vi "SW_Save_parameter_group_2.vi"(7 "Researcher name":string="Researcher", 8 "error in":errorcluster, 9 "Settings cluster in":T1={"Defaults"={"Default User"=0.0, "VISA Resource Name "="Tracker"}, "Recording and saving"={"Researcher name"="Researcher", "Name prefix"="Track", "Data post-processing"={"Filter type"=enum."Savitzky-Golay", "Length"=31, "Order"=3}, "Stop at"=0.0, "\"Stop at\" enabled"=FALSE, "Default save folder path"=path "", "Acquisition FPS"=enum."Max"}, "Geometry"={"Cage diameter, mm"=180, "Starting angle MIDFIELD"=0, "Starting angle BORDER"=0, "Radius, mm CENTER"=30, "Radius, mm MIDFIELD"=75, "N segments MIDFIELD"=2, "N segments BORDER"=4, "R-gap, mm"=0.0, "Bridge swap"=FALSE, "Bridge H. offset"=0.0, "Bridge V. offset"=0.0, "Twisted neck"=FALSE, "Alt. magn. orientation"=FALSE}, "IO parameters"={"IO general config."=12, "IO 1 configuration"=1, "IO 2 configuration"=1, "IO 3 configuration"=0, "IO 4 configuration"=0, "Activate ext. RS-232"=0, "IO inversion config."=0, "Sync capability"=1}, "Stimulus presets array"=[{"Event type"=0, "Dur., s"=0.0, "Stim., s"=0.0, "TTL out N"=1, "Set/Clear"=FALSE, "Stim. has been set"=FALSE}, {"Event type"=0, "Dur., s"=0.0, "Stim., s"=0.0, "TTL out N"=1, "Set/Clear"=FALSE, "Stim. has been set"=FALSE}, {"Event type"=0, "Dur., s"=0.0, "Stim., s"=0.0, "TTL out N"=1, "Set/Clear"=FALSE, "Stim. has been set"=FALSE}, {"Event type"=0, "Dur., s"=0.0, "Stim., s"=0.0, "TTL out N"=1, "Set/Clear"=FALSE, "Stim. has been set"=FALSE}, {"Event type"=0, "Dur., s"=0.0, "Stim., s"=0.0, "TTL out N"=1, "Set/Clear"=FALSE, "Stim. has been set"=FALSE}, {"Event type"=0, "Dur., s"=0.0, "Stim., s"=0.0, "TTL out N"=1, "Set/Clear"=FALSE, "Stim. has been set"=FALSE}, {"Event type"=0, "Dur., s"=0.0, "Stim., s"=0.0, "TTL out N"=1, "Set/Clear"=FALSE, "Stim. has been set"=FALSE}, {"Event type"=0, "Dur., s"=0.0, "Stim., s"=0.0, "TTL out N"=1, "Set/Clear"=FALSE, "Stim. has been set"=FALSE}, {"Event type"=0, "Dur., s"=0.0, "Stim., s"=0.0, "TTL out N"=1, "Set/Clear"=FALSE, "Stim. has been set"=FALSE}, {"Event type"=0, "Dur., s"=0.0, "Stim., s"=0.0, "TTL out N"=1, "Set/Clear"=FALSE, "Stim. has been set"=FALSE}, {"Event type"=0, "Dur., s"=0.0, "Stim., s"=0.0, "TTL out N"=1, "Set/Clear"=FALSE, "Stim. has been set"=FALSE}, {"Event type"=0, "Dur., s"=0.0, "Stim., s"=0.0, "TTL out N"=1, "Set/Clear"=FALSE, "Stim. has been set"=FALSE}, {"Event type"=0, "Dur., s"=0.0, "Stim., s"=0.0, "TTL out N"=1, "Set/Clear"=FALSE, "Stim. has been set"=FALSE}, {"Event type"=0, "Dur., s"=0.0, "Stim., s"=0.0, "TTL out N"=1, "Set/Clear"=FALSE, "Stim. has been set"=FALSE}], "Calibration parameters"={"Timing calibration sw/hw"=1.0, "True FPS"=80.0, "True frame time, s"=0.0125, "Disp. calibration info"=[]}, "Settings loaded OK"=FALSE} {"Calibration parameters"."True frame time, s" format="%.10g"; "Calibration parameters"."Disp. calibration info"."Speed, µl per ms" format="%.3g"; "Calibration parameters"."True FPS" format="%.10g"; "Calibration parameters"."Timing calibration sw/hw" format="%.10g"; "Stimulus presets array"."Event type" items=["Stay for N seconds"]; "Stimulus presets array"."TTL out N" items=["1"=1, "2"=2, "1+2"=3]; "Recording and saving"."Data post-processing"."Order" min=3 max=11 step=2; "Recording and saving"."Data post-processing"."Length" min=5 max=301 step=2; "Geometry"."Cage diameter, mm" scale=0.0..340.0}, 10 "Parameter group":T9="Defaults", 11 "Settings file refnum in":T10) -> (0 "error out":errorcluster, 2 "Saved OK?":bool, 3 "Settings file refnum out":T10)   [LabVIEW 2018, in "Tracker.lvlib"]
uses:
  Tracker.lvlib
  <vilib>/Utility/config.llb/Config Data RefNum.ctl
  Controls/CTL_Settings_parameters_groups.ctl
  Controls/CTL_Settings_cluster.ctl
  Controls/CTL_Filter_selector.ctl
  Controls/CTL_Acquisition_speed_selector.ctl
  Controls/CTL_Segmented_plot_parameters.ctl
  Controls/CTL_IO_params_cluster.ctl
  Controls/CTL_Single_stimulus_setting.ctl
  Controls/CTL_Calibration_parameters.ctl
  Controls/CTL_Dispenser_calibration_info.ctl
  <vilib>/Utility/config.llb/NI_LVConfig.lvlib
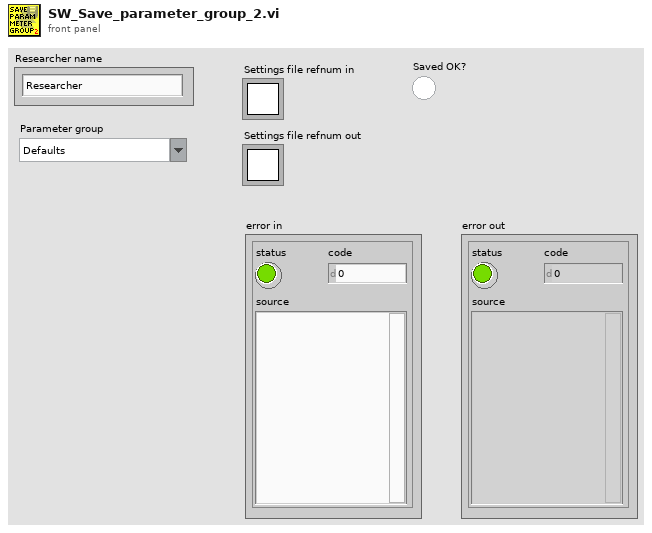
[diagram p1: front panel]
types:
  T1 = typedef "Tracker.lvlib/CTL_Settings_cluster.ctl" = cluster{"Defaults":cluster{"Default User":dbl, "VISA Resource Name ":string}, "Recording and saving":cluster{"Researcher name":string, "Name prefix":string, "Data post-processing":T2, "Stop at":dbl, "\"Stop at\" enabled":bool, "Default save folder path":path, "Acquisition FPS":T3}, "Geometry":T4, "IO parameters":T5, "Stimulus presets array":T6[], "Calibration parameters":T7, "Settings loaded OK":bool}
  T2 = typedef "Tracker.lvlib/CTL_Filter_selector.ctl" = cluster{"Filter type":enum16{"None", "Savitzky-Golay"}, "Length":i32, "Order":i32}
  T3 = typedef "Tracker.lvlib/CTL_Acquisition_speed_selector.ctl" = enum16{"Max", "Optimal", "Eco"}
  T4 = typedef "Tracker.lvlib/CTL_Segmented_plot_parameters.ctl" = cluster{"Cage diameter, mm":u16, "Starting angle MIDFIELD":i16, "Starting angle BORDER":i16, "Radius, mm CENTER":u16, "Radius, mm MIDFIELD":u16, "N segments MIDFIELD":u8, "N segments BORDER":u8, "R-gap, mm":sgl, "Bridge swap":bool, "Bridge H. offset":sgl, "Bridge V. offset":sgl, "Twisted neck":bool, "Alt. magn. orientation":bool}
  T5 = typedef "Tracker.lvlib/CTL_IO_params_cluster.ctl" = cluster{"IO general config.":u16, "IO 1 configuration":u16, "IO 2 configuration":u16, "IO 3 configuration":u16, "IO 4 configuration":u16, "Activate ext. RS-232":u16, "IO inversion config.":u16, "Sync capability":u8}
  T6 = typedef "Tracker.lvlib/CTL_Single_stimulus_setting.ctl" = cluster{"Event type":u16, "Dur., s":sgl, "Stim., s":sgl, "TTL out N":u16, "Set/Clear":bool, "Stim. has been set":bool}
  T7 = typedef "Tracker.lvlib/CTL_Calibration_parameters.ctl" = cluster{"Timing calibration sw/hw":dbl, "True FPS":dbl, "True frame time, s":dbl, "Disp. calibration info":T8}
  T8 = typedef "Tracker.lvlib/CTL_Dispenser_calibration_info.ctl" = cluster{"Channel":u8, "Speed, µl per ms":dbl}[]
  T9 = typedef "Tracker.lvlib/CTL_Settings_parameters_groups.ctl" = string
  T10 = typedef "NI_LVConfig.lvlib/Config Data RefNum.ctl" = refnum<k1>
  T11 = cluster{"Default User":dbl, "VISA Resource Name ":string}
  T12 = cluster{"Researcher name":string, "Name prefix":string, "Data post-processing":T2, "Stop at":dbl, "\"Stop at\" enabled":bool, "Default save folder path":path, "Acquisition FPS":T3}
  T13 = cluster{"Stimulus presets array[0]":T6, "Stimulus presets array[1]":T6, "Stimulus presets array[2]":T6, "Stimulus presets array[3]":T6, "Stimulus presets array[4]":T6, "Stimulus presets array[5]":T6, "Stimulus presets array[6]":T6, "Stimulus presets array[7]":T6, "Stimulus presets array[8]":T6, "Stimulus presets array[9]":T6, "Stimulus presets array[10]":T6, "Stimulus presets array[11]":T6, "Stimulus presets array[12]":T6, "Stimulus presets array[13]":T6}
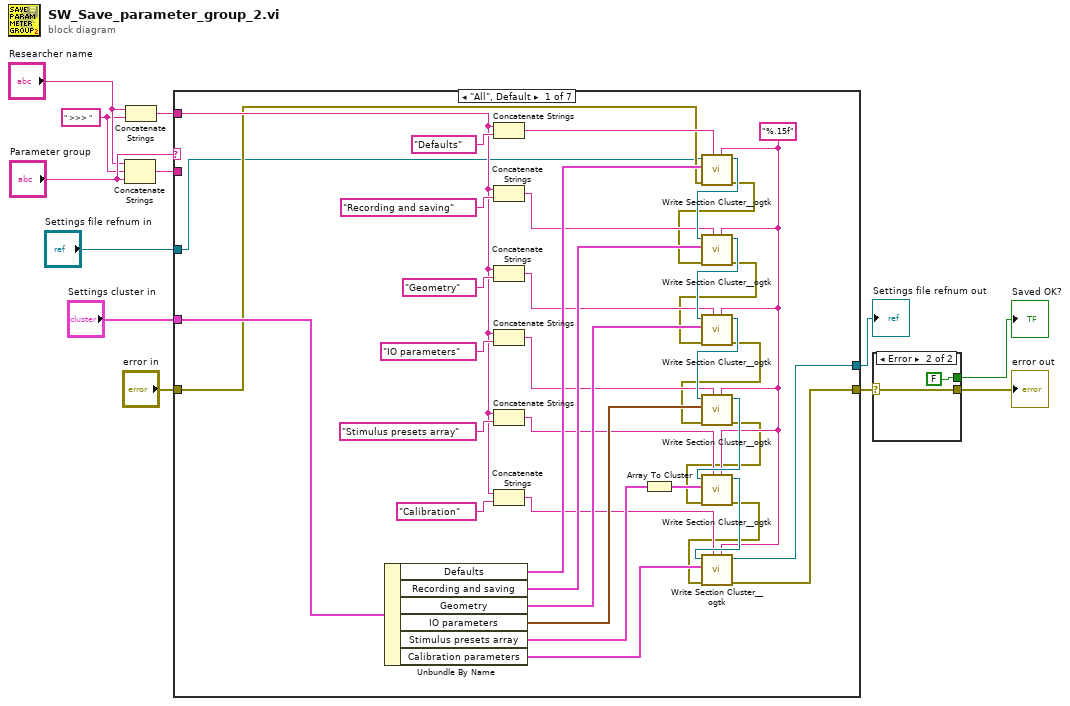
[diagram p0: block diagram]
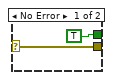
[diagram p2: hidden frame]
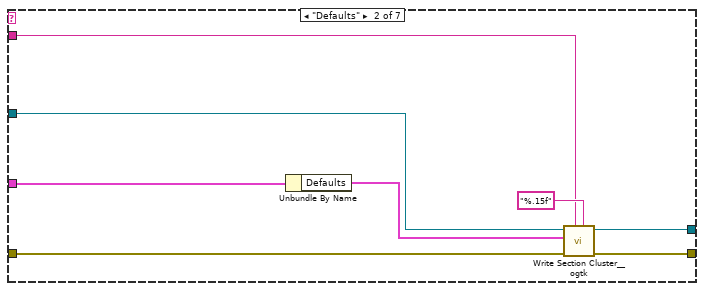
[diagram p3: hidden frame]
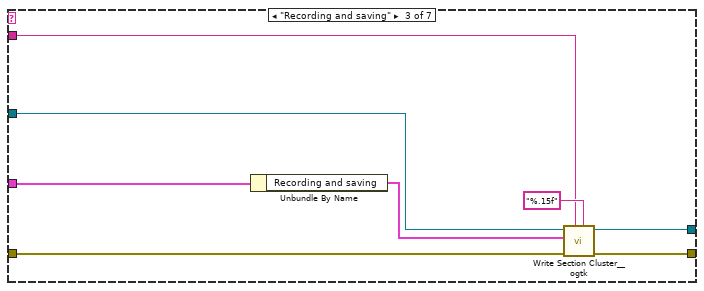
[diagram p4: hidden frame]
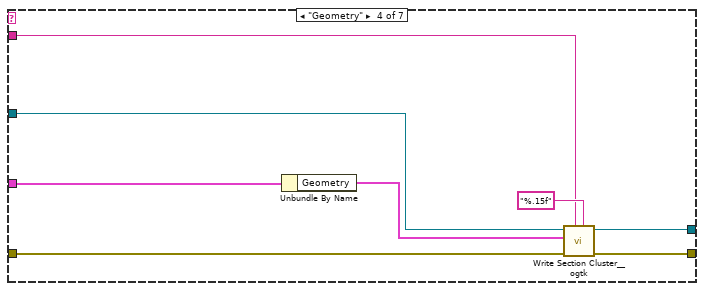
[diagram p5: hidden frame]
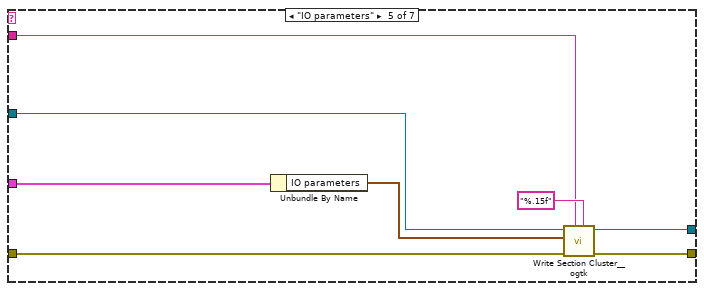
[diagram p6: hidden frame]
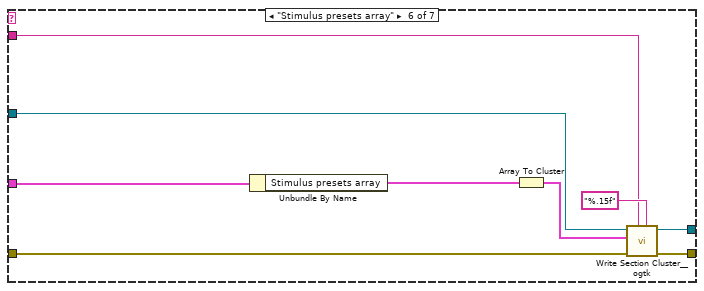
[diagram p7: hidden frame]
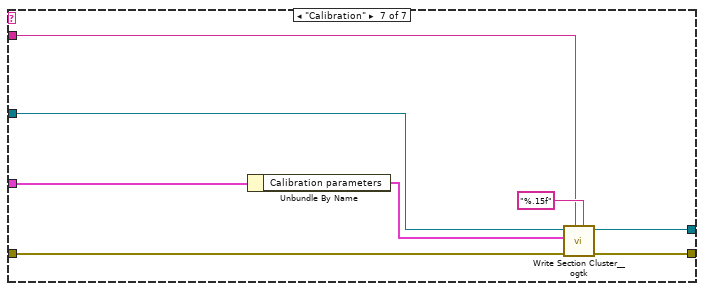
[diagram p8: hidden frame]
diagram:
  w2 = " >>> " ("string")
  n1 = Concatenate Strings("Researcher name", w2, "Parameter group") -> (w10:string)
  n2 = Concatenate Strings("Researcher name", w2) -> (w1:string)
  n3 = case shown="\"All\", Default" "Parameter group" {
    tunnel: "Settings cluster in" -> [w48 w54 w62 w70 w78 w87 w95]
    tunnel: w10 -> [_ w55 w63 w71 w79 w88 w96]
    tunnel: "error in" -> [w20 w53 w61 w69 w77 w86 w94]
    tunnel: "Settings file refnum in" -> [w19 w52 w60 w68 w76 w85 w93]
    tunnel: [w21 w51 w59 w67 w75 w84 w92] -> w8
    tunnel: [w13 w50 w58 w66 w74 w83 w91] -> w7
    tunnel: w1 -> [w24 _ _ _ _ _ _]
    frame "All", Default {
      w22 = "%.15f" ("float number format (optional)")
      n4 = Unbundle By Name(w48) -> ("Defaults"=w45:T11, "Recording and saving"=w41:T12, "Geometry"=w38:T4, "IO parameters"=w33:T5, "Stimulus presets array"=w28:T6[], "Calibration parameters"=w26:T7)
      n5 = Concatenate Strings(w24, T9 "Defaults" ("Parameter group")) -> (w47:string)
      n6 = Concatenate Strings(w24, T9 "Recording and saving" ("Parameter group")) -> (w42:string)
      n7 = Concatenate Strings(w24, T9 "Geometry" ("Parameter group")) -> (w37:string)
      n8 = Concatenate Strings(w24, T9 "IO parameters" ("Parameter group")) -> (w34:string)
      n9 = Concatenate Strings(w24, T9 "Stimulus presets array" ("Parameter group")) -> (w29:string)
      n10 = Concatenate Strings(w24, T9 "Calibration" ("Parameter group")) -> (w23:string)
      n11 = Array To Cluster(array=w28) -> (cluster=w27:T13)
      n12 = call <userlib>:"Write Section Cluster__ogtk.vi"("float number format (optional)"=w22, "section (optional)"=w47, "error in (no error)"=w20, "Section Formatted Cluster"=w45, "refnum"=w19) -> ("error out"=w18:errorcluster, "dup refnum"=w44:T10)  [unwired: 5 in]
      n13 = call <userlib>:"Write Section Cluster__ogtk.vi"("float number format (optional)"=w22, "section (optional)"=w42, "error in (no error)"=w18, "Section Formatted Cluster"=w41, "refnum"=w44) -> ("error out"=w17:errorcluster, "dup refnum"=w40:T10)  [unwired: 5 in]
      n14 = call <userlib>:"Write Section Cluster__ogtk.vi"("float number format (optional)"=w22, "section (optional)"=w37, "error in (no error)"=w17, "Section Formatted Cluster"=w38, "refnum"=w40) -> ("error out"=w16:errorcluster, "dup refnum"=w36:T10)  [unwired: 5 in]
      n15 = call <userlib>:"Write Section Cluster__ogtk.vi"("float number format (optional)"=w22, "section (optional)"=w34, "error in (no error)"=w16, "Section Formatted Cluster"=w33, "refnum"=w36) -> ("error out"=w15:errorcluster, "dup refnum"=w32:T10)  [unwired: 5 in]
      n16 = call <userlib>:"Write Section Cluster__ogtk.vi"("float number format (optional)"=w22, "section (optional)"=w29, "error in (no error)"=w15, "Section Formatted Cluster"=w27, "refnum"=w32) -> ("error out"=w14:errorcluster, "dup refnum"=w31:T10)  [unwired: 5 in]
      n17 = call <userlib>:"Write Section Cluster__ogtk.vi"("float number format (optional)"=w22, "section (optional)"=w23, "error in (no error)"=w14, "Section Formatted Cluster"=w26, "refnum"=w31) -> ("error out"=w13:errorcluster, "dup refnum"=w21:T10)  [unwired: 5 in]
    }
    frame "Defaults" {
      n18 = Unbundle By Name(w54) -> ("Defaults"=w49:T11)
      n19 = call <userlib>:"Write Section Cluster__ogtk.vi"("float number format (optional)"="%.15f", "section (optional)"=w55, "error in (no error)"=w53, "Section Formatted Cluster"=w49, "refnum"=w52) -> ("error out"=w50:errorcluster, "dup refnum"=w51:T10)  [unwired: 5 in]
    }
    frame "Recording and saving" {
      n20 = Unbundle By Name(w62) -> ("Recording and saving"=w57:T12)
      n21 = call <userlib>:"Write Section Cluster__ogtk.vi"("float number format (optional)"="%.15f", "section (optional)"=w63, "error in (no error)"=w61, "Section Formatted Cluster"=w57, "refnum"=w60) -> ("error out"=w58:errorcluster, "dup refnum"=w59:T10)  [unwired: 5 in]
    }
    frame "Geometry" {
      n22 = Unbundle By Name(w70) -> ("Geometry"=w65:T4)
      n23 = call <userlib>:"Write Section Cluster__ogtk.vi"("float number format (optional)"="%.15f", "section (optional)"=w71, "error in (no error)"=w69, "Section Formatted Cluster"=w65, "refnum"=w68) -> ("error out"=w66:errorcluster, "dup refnum"=w67:T10)  [unwired: 5 in]
    }
    frame "IO parameters" {
      n24 = Unbundle By Name(w78) -> ("IO parameters"=w73:T5)
      n25 = call <userlib>:"Write Section Cluster__ogtk.vi"("float number format (optional)"="%.15f", "section (optional)"=w79, "error in (no error)"=w77, "Section Formatted Cluster"=w73, "refnum"=w76) -> ("error out"=w74:errorcluster, "dup refnum"=w75:T10)  [unwired: 5 in]
    }
    frame "Stimulus presets array" {
      n26 = Unbundle By Name(w87) -> ("Stimulus presets array"=w82:T6[])
      n27 = Array To Cluster(array=w82) -> (cluster=w81:T13)
      n28 = call <userlib>:"Write Section Cluster__ogtk.vi"("float number format (optional)"="%.15f", "section (optional)"=w88, "error in (no error)"=w86, "Section Formatted Cluster"=w81, "refnum"=w85) -> ("error out"=w83:errorcluster, "dup refnum"=w84:T10)  [unwired: 5 in]
    }
    frame "Calibration" {
      n29 = Unbundle By Name(w95) -> ("Calibration parameters"=w90:T7)
      n30 = call <userlib>:"Write Section Cluster__ogtk.vi"("float number format (optional)"="%.15f", "section (optional)"=w96, "error in (no error)"=w94, "Section Formatted Cluster"=w90, "refnum"=w93) -> ("error out"=w91:errorcluster, "dup refnum"=w92:T10)  [unwired: 5 in]
    }
  }
  "Settings file refnum out" <- w8
  n31 = case shown="Error" w7 {
    selector: w7 -> [w99 w101]
    tunnel: [w99 w101] -> w6
    tunnel: [TRUE FALSE] -> w5
    frame No Error {
    }
    frame Error {
    }
  }
  "error out" <- w6
  "Saved OK?" <- w5
